vi "Get Data.vi"(8 "error in":errorcluster, 11 "Cfg Dev in":refnum<class "PPT.lvclass">) -> (0 "error out":errorcluster, 2 "Data":refnum<class "Data.lvclass">, 3 "Cfg Dev out":refnum<class "PPT.lvclass">)   [LabVIEW 2014, in "PPT.lvclass"]
doc: "Retrieves pressure and temperature in a SGL_Array Data object. Temperature is obtained via the 'T1' command and the Pressure via the 'P1' command."
uses:
  PPT.lvclass
  Reusable/Data/Data.lvclass
  Reusable/Data/Array Data/Single 1-D/Single_Array.lvclass
  Get Pressure.vi
  Get Temperature.vi
  Reusable/Data/Array Data/Single 1-D/Write Data.vi
  Reusable/Data/Write measTime.vi
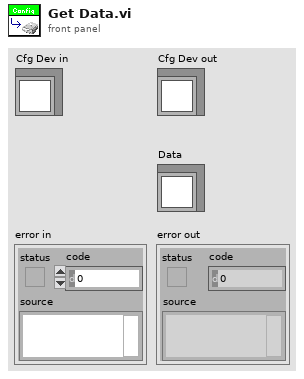
[diagram p1: front panel]
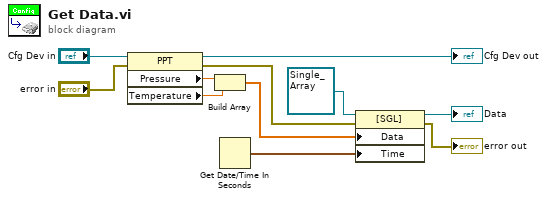
[diagram p0: block diagram]
diagram:
  n1 = property class="PPT"(reference="Cfg Dev in", error in="error in") -> (reference out=→"Cfg Dev out":refnum<class "PPT.lvclass">, error out=w1:errorcluster, "Pressure"=w5:dbl, "Temperature"=w4:dbl)
  n2 = Build Array(w5, w4) -> (w10:dbl[])
  n3 = Get Date/Time In Seconds() -> (seconds since 1Jan1904=w9:timestamp)
  n4 = property class="[SGL]"(reference=refnum<class "Single_Array.lvclass"> refnum ("Base Data Lib:[SGL]"), error in=w1, "Data"=w10, "Time"=w9) -> (reference out=→"Data":refnum<class "Single_Array.lvclass">, error out=→"error out":errorcluster)
